vi "main_rek.vi"() -> ()   [LabVIEW 2017]
panel:
  out "StringOut":string
  in  "Numeric":i32
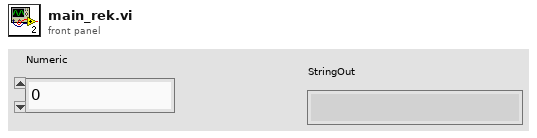
[diagram p1: front panel]
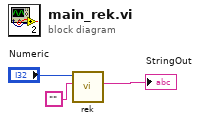
[diagram p0: block diagram]
diagram:
  n1 = call "rek.vi"("StringIn"="", "Numeric"="Numeric") -> ("StringOut"=→"StringOut":string)  [unwired: 9 in]
